vi "DeviceDiscovery.vi"() -> (2 "deviceInfo out":T1, 3 "Ip":string)   [LabVIEW 2019]
uses:
  EmergentCameraC/EmergentCameraC.lvlib
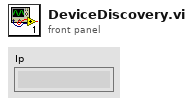
[diagram p1: front panel]
types:
  T1 = cluster{"specVersionMajor":u16, "specVersionMinor":u16, "deviceMode":u32, "macAddress[0]":i8, "macAddress[1]":i8, "macAddress[2]":i8, "macAddress[3]":i8, "macAddress[4]":i8, "macAddress[5]":i8, "macAddress[6]":i8, "macAddress[7]":i8, "macAddress[8]":i8, "macAddress[9]":i8, "macAddress[10]":i8, "macAddress[11]":i8, "macAddress[12]":i8, "macAddress[13]":i8, "macAddress[14]":i8, "macAddress[15]":i8, "macAddress[16]":i8, "macAddress[17]":i8, "@dummy control@":i8, "@dummy control@":i8, "ipConfigOptions":u32, "ipConfigCurrent":u32, "currentIp[0]":i8, "currentIp[1]":i8, "currentIp[2]":i8, "currentIp[3]":i8, "currentIp[4]":i8, "currentIp[5]":i8, "currentIp[6]":i8, "currentIp[7]":i8, "currentIp[8]":i8, "currentIp[9]":i8, "currentIp[10]":i8, "currentIp[11]":i8, "currentIp[12]":i8, "currentIp[13]":i8, "currentIp[14]":i8, "currentIp[15]":i8, "currentSubnetMask[0]":i8, "currentSubnetMask[1]":i8, "currentSubnetMask[2]":i8, "currentSubnetMask[3]":i8, "currentSubnetMask[4]":i8, "currentSubnetMask[5]":i8, "currentSubnetMask[6]":i8, "currentSubnetMask[7]":i8, "currentSubnetMask[8]":i8, "currentSubnetMask[9]":i8, "currentSubnetMask[10]":i8, "currentSubnetMask[11]":i8, "currentSubnetMask[12]":i8, "currentSubnetMask[13]":i8, "currentSubnetMask[14]":i8, "currentSubnetMask[15]":i8, "defaultGateway[0]":i8, "defaultGateway[1]":i8, "defaultGateway[2]":i8, "defaultGateway[3]":i8, "defaultGateway[4]":i8, "defaultGateway[5]":i8, "defaultGateway[6]":i8, "defaultGateway[7]":i8, "defaultGateway[8]":i8, "defaultGateway[9]":i8, "defaultGateway[10]":i8, "defaultGateway[11]":i8, "defaultGateway[12]":i8, "defaultGateway[13]":i8, "defaultGateway[14]":i8, "defaultGateway[15]":i8, "manufacturerName[0]":i8, "manufacturerName[1]":i8, "manufacturerName[2]":i8, "manufacturerName[3]":i8, "manufacturerName[4]":i8, "manufacturerName[5]":i8, "manufacturerName[6]":i8, "manufacturerName[7]":i8, "manufacturerName[8]":i8, "manufacturerName[9]":i8, "manufacturerName[10]":i8, "manufacturerName[11]":i8, "manufacturerName[12]":i8, "manufacturerName[13]":i8, "manufacturerName[14]":i8, "manufacturerName[15]":i8, "manufacturerName[16]":i8, "manufacturerName[17]":i8, "manufacturerName[18]":i8, "manufacturerName[19]":i8, "manufacturerName[20]":i8, "manufacturerName[21]":i8, "manufacturerName[22]":i8, "manufacturerName[23]":i8, "manufacturerName[24]":i8, "manufacturerName[25]":i8, "manufacturerName[26]":i8, "manufacturerName[27]":i8, "manufacturerName[28]":i8, "manufacturerName[29]":i8, "manufacturerName[30]":i8, "manufacturerName[31]":i8, "modelName[0]":i8, "modelName[1]":i8, "modelName[2]":i8, "modelName[3]":i8, "modelName[4]":i8, "modelName[5]":i8, "modelName[6]":i8, "modelName[7]":i8, "modelName[8]":i8, "modelName[9]":i8, "modelName[10]":i8, "modelName[11]":i8, "modelName[12]":i8, "modelName[13]":i8, "modelName[14]":i8, "modelName[15]":i8, "modelName[16]":i8, "modelName[17]":i8, "modelName[18]":i8, "modelName[19]":i8, "modelName[20]":i8, "modelName[21]":i8, "modelName[22]":i8, "modelName[23]":i8, "modelName[24]":i8, "modelName[25]":i8, "modelName[26]":i8, "modelName[27]":i8, "modelName[28]":i8, "modelName[29]":i8, "modelName[30]":i8, "modelName[31]":i8, "deviceVersion[0]":i8, "deviceVersion[1]":i8, "deviceVersion[2]":i8, "deviceVersion[3]":i8, "deviceVersion[4]":i8, "deviceVersion[5]":i8, "deviceVersion[6]":i8, "deviceVersion[7]":i8, "deviceVersion[8]":i8, "deviceVersion[9]":i8, "deviceVersion[10]":i8, "deviceVersion[11]":i8, "deviceVersion[12]":i8, "deviceVersion[13]":i8, "deviceVersion[14]":i8, "deviceVersion[15]":i8, "deviceVersion[16]":i8, "deviceVersion[17]":i8, "deviceVersion[18]":i8, "deviceVersion[19]":i8, "deviceVersion[20]":i8, "deviceVersion[21]":i8, "deviceVersion[22]":i8, "deviceVersion[23]":i8, "deviceVersion[24]":i8, "deviceVersion[25]":i8, "deviceVersion[26]":i8, "deviceVersion[27]":i8, "deviceVersion[28]":i8, "deviceVersion[29]":i8, "deviceVersion[30]":i8, "deviceVersion[31]":i8, "manufacturerSpecifiedInfo[0]":i8, "manufacturerSpecifiedInfo[1]":i8, "manufacturerSpecifiedInfo[2]":i8, "manufacturerSpecifiedInfo[3]":i8, "manufacturerSpecifiedInfo[4]":i8, "manufacturerSpecifiedInfo[5]":i8, "manufacturerSpecifiedInfo[6]":i8, "manufacturerSpecifiedInfo[7]":i8, "manufacturerSpecifiedInfo[8]":i8, "manufacturerSpecifiedInfo[9]":i8, "manufacturerSpecifiedInfo[10]":i8, "manufacturerSpecifiedInfo[11]":i8, "manufacturerSpecifiedInfo[12]":i8, "manufacturerSpecifiedInfo[13]":i8, "manufacturerSpecifiedInfo[14]":i8, "manufacturerSpecifiedInfo[15]":i8, "manufacturerSpecifiedInfo[16]":i8, "manufacturerSpecifiedInfo[17]":i8, "manufacturerSpecifiedInfo[18]":i8, "manufacturerSpecifiedInfo[19]":i8, "manufacturerSpecifiedInfo[20]":i8, "manufacturerSpecifiedInfo[21]":i8, "manufacturerSpecifiedInfo[22]":i8, "manufacturerSpecifiedInfo[23]":i8, "manufacturerSpecifiedInfo[24]":i8, "manufacturerSpecifiedInfo[25]":i8, "manufacturerSpecifiedInfo[26]":i8, "manufacturerSpecifiedInfo[27]":i8, "manufacturerSpecifiedInfo[28]":i8, "manufacturerSpecifiedInfo[29]":i8, "manufacturerSpecifiedInfo[30]":i8, "manufacturerSpecifiedInfo[31]":i8, "manufacturerSpecifiedInfo[32]":i8, "manufacturerSpecifiedInfo[33]":i8, "manufacturerSpecifiedInfo[34]":i8, "manufacturerSpecifiedInfo[35]":i8, "manufacturerSpecifiedInfo[36]":i8, "manufacturerSpecifiedInfo[37]":i8, "manufacturerSpecifiedInfo[38]":i8, "manufacturerSpecifiedInfo[39]":i8, "manufacturerSpecifiedInfo[40]":i8, "manufacturerSpecifiedInfo[41]":i8, "manufacturerSpecifiedInfo[42]":i8, "manufacturerSpecifiedInfo[43]":i8, "manufacturerSpecifiedInfo[44]":i8, "manufacturerSpecifiedInfo[45]":i8, "manufacturerSpecifiedInfo[46]":i8, "manufacturerSpecifiedInfo[47]":i8, "serialNumber[0]":i8, "serialNumber[1]":i8, "serialNumber[2]":i8, "serialNumber[3]":i8, "serialNumber[4]":i8, "serialNumber[5]":i8, "serialNumber[6]":i8, "serialNumber[7]":i8, "serialNumber[8]":i8, "serialNumber[9]":i8, "serialNumber[10]":i8, "serialNumber[11]":i8, "serialNumber[12]":i8, "serialNumber[13]":i8, "serialNumber[14]":i8, "serialNumber[15]":i8, "userDefinedName[0]":i8, "userDefinedName[1]":i8, "userDefinedName[2]":i8, "userDefinedName[3]":i8, "userDefinedName[4]":i8, "userDefinedName[5]":i8, "userDefinedName[6]":i8, "userDefinedName[7]":i8, "userDefinedName[8]":i8, "userDefinedName[9]":i8, "userDefinedName[10]":i8, "userDefinedName[11]":i8, "userDefinedName[12]":i8, "userDefinedName[13]":i8, "userDefinedName[14]":i8, "userDefinedName[15]":i8, "ip4Address[0]":i8, "ip4Address[1]":i8, "ip4Address[2]":i8, "ip4Address[3]":i8, "ip4Address[4]":i8, "ip4Address[5]":i8, "ip4Address[6]":i8, "ip4Address[7]":i8, "ip4Address[8]":i8, "ip4Address[9]":i8, "ip4Address[10]":i8, "ip4Address[11]":i8, "ip4Address[12]":i8, "ip4Address[13]":i8, "ip4Address[14]":i8, "ip4Address[15]":i8, "ip4AddressBroadcast[0]":i8, "ip4AddressBroadcast[1]":i8, "ip4AddressBroadcast[2]":i8, "ip4AddressBroadcast[3]":i8, "ip4AddressBroadcast[4]":i8, "ip4AddressBroadcast[5]":i8, "ip4AddressBroadcast[6]":i8, "ip4AddressBroadcast[7]":i8, "ip4AddressBroadcast[8]":i8, "ip4AddressBroadcast[9]":i8, "ip4AddressBroadcast[10]":i8, "ip4AddressBroadcast[11]":i8, "ip4AddressBroadcast[12]":i8, "ip4AddressBroadcast[13]":i8, "ip4AddressBroadcast[14]":i8, "ip4AddressBroadcast[15]":i8, "friendlyName[0]":i8, "friendlyName[1]":i8, "friendlyName[2]":i8, "friendlyName[3]":i8, "friendlyName[4]":i8, "friendlyName[5]":i8, "friendlyName[6]":i8, "friendlyName[7]":i8, "friendlyName[8]":i8, "friendlyName[9]":i8, "friendlyName[10]":i8, "friendlyName[11]":i8, "friendlyName[12]":i8, "friendlyName[13]":i8, "friendlyName[14]":i8, "friendlyName[15]":i8, "friendlyName[16]":i8, "friendlyName[17]":i8, "friendlyName[18]":i8, "friendlyName[19]":i8, "friendlyName[20]":i8, "friendlyName[21]":i8, "friendlyName[22]":i8, "friendlyName[23]":i8, "friendlyName[24]":i8, "friendlyName[25]":i8, "friendlyName[26]":i8, "friendlyName[27]":i8, "friendlyName[28]":i8, "friendlyName[29]":i8, "friendlyName[30]":i8, "friendlyName[31]":i8, "friendlyName[32]":i8, "friendlyName[33]":i8, "friendlyName[34]":i8, "friendlyName[35]":i8, "friendlyName[36]":i8, "friendlyName[37]":i8, "friendlyName[38]":i8, "friendlyName[39]":i8, "friendlyName[40]":i8, "friendlyName[41]":i8, "friendlyName[42]":i8, "friendlyName[43]":i8, "friendlyName[44]":i8, "friendlyName[45]":i8, "friendlyName[46]":i8, "friendlyName[47]":i8, "friendlyName[48]":i8, "friendlyName[49]":i8, "friendlyName[50]":i8, "friendlyName[51]":i8, "friendlyName[52]":i8, "friendlyName[53]":i8, "friendlyName[54]":i8, "friendlyName[55]":i8, "friendlyName[56]":i8, "friendlyName[57]":i8, "friendlyName[58]":i8, "friendlyName[59]":i8, "friendlyName[60]":i8, "friendlyName[61]":i8, "friendlyName[62]":i8, "friendlyName[63]":i8, "friendlyName[64]":i8, "friendlyName[65]":i8, "friendlyName[66]":i8, "friendlyName[67]":i8, "friendlyName[68]":i8, "friendlyName[69]":i8, "friendlyName[70]":i8, "friendlyName[71]":i8, "friendlyName[72]":i8, "friendlyName[73]":i8, "friendlyName[74]":i8, "friendlyName[75]":i8, "friendlyName[76]":i8, "friendlyName[77]":i8, "friendlyName[78]":i8, "friendlyName[79]":i8, "friendlyName[80]":i8, "friendlyName[81]":i8, "friendlyName[82]":i8, "friendlyName[83]":i8, "friendlyName[84]":i8, "friendlyName[85]":i8, "friendlyName[86]":i8, "friendlyName[87]":i8, "friendlyName[88]":i8, "friendlyName[89]":i8, "friendlyName[90]":i8, "friendlyName[91]":i8, "friendlyName[92]":i8, "friendlyName[93]":i8, "friendlyName[94]":i8, "friendlyName[95]":i8, "friendlyName[96]":i8, "friendlyName[97]":i8, "friendlyName[98]":i8, "friendlyName[99]":i8, "friendlyName[100]":i8, "friendlyName[101]":i8, "friendlyName[102]":i8, "friendlyName[103]":i8, "friendlyName[104]":i8, "friendlyName[105]":i8, "friendlyName[106]":i8, "friendlyName[107]":i8, "friendlyName[108]":i8, "friendlyName[109]":i8, "friendlyName[110]":i8, "friendlyName[111]":i8, "friendlyName[112]":i8, "friendlyName[113]":i8, "friendlyName[114]":i8, "friendlyName[115]":i8, "friendlyName[116]":i8, "friendlyName[117]":i8, "friendlyName[118]":i8, "friendlyName[119]":i8, "friendlyName[120]":i8, "friendlyName[121]":i8, "friendlyName[122]":i8, "friendlyName[123]":i8, "friendlyName[124]":i8, "friendlyName[125]":i8, "friendlyName[126]":i8, "friendlyName[127]":i8, "description[0]":i8, "description[1]":i8, "description[2]":i8, "description[3]":i8, "description[4]":i8, "description[5]":i8, "description[6]":i8, "description[7]":i8, "description[8]":i8, "description[9]":i8, "description[10]":i8, "description[11]":i8, "description[12]":i8, "description[13]":i8, "description[14]":i8, "description[15]":i8, "description[16]":i8, "description[17]":i8, "description[18]":i8, "description[19]":i8, "description[20]":i8, "description[21]":i8, "description[22]":i8, "description[23]":i8, "description[24]":i8, "description[25]":i8, "description[26]":i8, "description[27]":i8, "description[28]":i8, "description[29]":i8, "description[30]":i8, "description[31]":i8, "description[32]":i8, "description[33]":i8, "description[34]":i8, "description[35]":i8, "description[36]":i8, "description[37]":i8, "description[38]":i8, "description[39]":i8, "description[40]":i8, "description[41]":i8, "description[42]":i8, "description[43]":i8, "description[44]":i8, "description[45]":i8, "description[46]":i8, "description[47]":i8, "description[48]":i8, "description[49]":i8, "description[50]":i8, "description[51]":i8, "description[52]":i8, "description[53]":i8, "description[54]":i8, "description[55]":i8, "description[56]":i8, "description[57]":i8, "description[58]":i8, "description[59]":i8, "description[60]":i8, "description[61]":i8, "description[62]":i8, "description[63]":i8, "description[64]":i8, "description[65]":i8, "description[66]":i8, "description[67]":i8, "description[68]":i8, "description[69]":i8, "description[70]":i8, "description[71]":i8, "description[72]":i8, "description[73]":i8, "description[74]":i8, "description[75]":i8, "description[76]":i8, "description[77]":i8, "description[78]":i8, "description[79]":i8, "description[80]":i8, "description[81]":i8, "description[82]":i8, "description[83]":i8, "description[84]":i8, "description[85]":i8, "description[86]":i8, "description[87]":i8, "description[88]":i8, "description[89]":i8, "description[90]":i8, "description[91]":i8, "description[92]":i8, "description[93]":i8, "description[94]":i8, "description[95]":i8, "description[96]":i8, "description[97]":i8, "description[98]":i8, "description[99]":i8, "description[100]":i8, "description[101]":i8, "description[102]":i8, "description[103]":i8, "description[104]":i8, "description[105]":i8, "description[106]":i8, "description[107]":i8, "description[108]":i8, "description[109]":i8, "description[110]":i8, "description[111]":i8, "description[112]":i8, "description[113]":i8, "description[114]":i8, "description[115]":i8, "description[116]":i8, "description[117]":i8, "description[118]":i8, "description[119]":i8, "description[120]":i8, "description[121]":i8, "description[122]":i8, "description[123]":i8, "description[124]":i8, "description[125]":i8, "description[126]":i8, "description[127]":i8, "adapterName[0]":i8, "adapterName[1]":i8, "adapterName[2]":i8, "adapterName[3]":i8, "adapterName[4]":i8, "adapterName[5]":i8, "adapterName[6]":i8, "adapterName[7]":i8, "adapterName[8]":i8, "adapterName[9]":i8, "adapterName[10]":i8, "adapterName[11]":i8, "adapterName[12]":i8, "adapterName[13]":i8, "adapterName[14]":i8, "adapterName[15]":i8, "adapterName[16]":i8, "adapterName[17]":i8, "adapterName[18]":i8, "adapterName[19]":i8, "adapterName[20]":i8, "adapterName[21]":i8, "adapterName[22]":i8, "adapterName[23]":i8, "adapterName[24]":i8, "adapterName[25]":i8, "adapterName[26]":i8, "adapterName[27]":i8, "adapterName[28]":i8, "adapterName[29]":i8, "adapterName[30]":i8, "adapterName[31]":i8, "adapterName[32]":i8, "adapterName[33]":i8, "adapterName[34]":i8, "adapterName[35]":i8, "adapterName[36]":i8, "adapterName[37]":i8, "adapterName[38]":i8, "adapterName[39]":i8, "adapterName[40]":i8, "adapterName[41]":i8, "adapterName[42]":i8, "adapterName[43]":i8, "adapterName[44]":i8, "adapterName[45]":i8, "adapterName[46]":i8, "adapterName[47]":i8, "adapterName[48]":i8, "adapterName[49]":i8, "adapterName[50]":i8, "adapterName[51]":i8, "adapterName[52]":i8, "adapterName[53]":i8, "adapterName[54]":i8, "adapterName[55]":i8, "adapterName[56]":i8, "adapterName[57]":i8, "adapterName[58]":i8, "adapterName[59]":i8, "adapterName[60]":i8, "adapterName[61]":i8, "adapterName[62]":i8, "adapterName[63]":i8, "adapterName[64]":i8, "adapterName[65]":i8, "adapterName[66]":i8, "adapterName[67]":i8, "adapterName[68]":i8, "adapterName[69]":i8, "adapterName[70]":i8, "adapterName[71]":i8, "adapterName[72]":i8, "adapterName[73]":i8, "adapterName[74]":i8, "adapterName[75]":i8, "adapterName[76]":i8, "adapterName[77]":i8, "adapterName[78]":i8, "adapterName[79]":i8, "adapterName[80]":i8, "adapterName[81]":i8, "adapterName[82]":i8, "adapterName[83]":i8, "adapterName[84]":i8, "adapterName[85]":i8, "adapterName[86]":i8, "adapterName[87]":i8, "adapterName[88]":i8, "adapterName[89]":i8, "adapterName[90]":i8, "adapterName[91]":i8, "adapterName[92]":i8, "adapterName[93]":i8, "adapterName[94]":i8, "adapterName[95]":i8, "adapterName[96]":i8, "adapterName[97]":i8, "adapterName[98]":i8, "adapterName[99]":i8, "adapterName[100]":i8, "adapterName[101]":i8, "adapterName[102]":i8, "adapterName[103]":i8, "adapterName[104]":i8, "adapterName[105]":i8, "adapterName[106]":i8, "adapterName[107]":i8, "adapterName[108]":i8, "adapterName[109]":i8, "adapterName[110]":i8, "adapterName[111]":i8, "adapterName[112]":i8, "adapterName[113]":i8, "adapterName[114]":i8, "adapterName[115]":i8, "adapterName[116]":i8, "adapterName[117]":i8, "adapterName[118]":i8, "adapterName[119]":i8, "adapterName[120]":i8, "adapterName[121]":i8, "adapterName[122]":i8, "adapterName[123]":i8, "adapterName[124]":i8, "adapterName[125]":i8, "adapterName[126]":i8, "adapterName[127]":i8, "vendorID":u32, "@dummy control@":i8, "@dummy control@":i8, "@dummy control@":i8, "@dummy control@":i8, "@dummy control@":i8, "@dummy control@":i8, "@dummy control@":i8, "@dummy control@":i8, "name":u64, "fullName":u64, "mtu":u32}
  T2 = cluster{"currentIp[0]":i8, "currentIp[1]":i8, "currentIp[2]":i8, "currentIp[3]":i8, "currentIp[4]":i8, "currentIp[5]":i8, "currentIp[6]":i8, "currentIp[7]":i8, "currentIp[8]":i8, "currentIp[9]":i8, "currentIp[10]":i8, "currentIp[11]":i8, "currentIp[12]":i8, "currentIp[13]":i8, "currentIp[14]":i8, "currentIp[15]":i8}
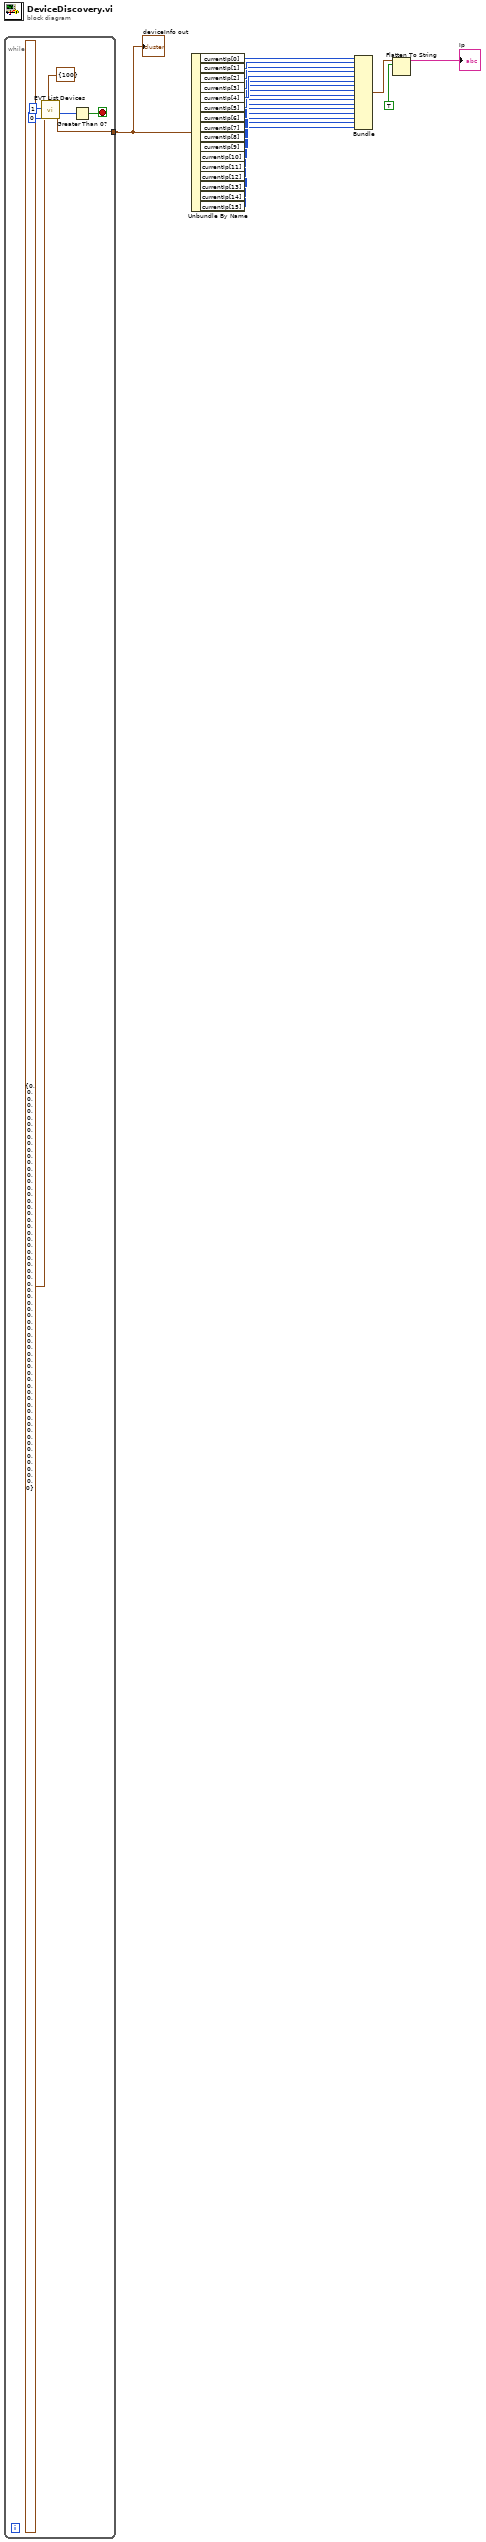
[diagram p0: block diagram]
diagram:
  n1 = while {
    tunnel: [w24] -> w2
    stop <- w23 stop-if-true
    n2 = call "EVT List Devices.vi"("settings"=cluster{"timeout":i32} {"timeout"=100}, "actualNum"=u32 0, "bufSize"=u32 1, "deviceInfo"=T1 {"specVersionMajor"=0, "specVersionMinor"=0, "deviceMode"=0, "macAddress[0]"=0, "macAddress[1]"=0, "macAddress[2]"=0, "macAddress[3]"=0, "macAddress[4]"=0, "macAddress[5]"=0, "macAddress[6]"=0, "macAddress[7]"=0, "macAddress[8]"=0, "macAddress[9]"=0, "macAddress[10]"=0, "macAddress[11]"=0, "macAddress[12]"=0, "macAddress[13]"=0, "macAddress[14]"=0, "macAddress[15]"=0, "macAddress[16]"=0, "macAddress[17]"=0, "@dummy control@"=0, "@dummy control@"=0, "ipConfigOptions"=0, "ipConfigCurrent"=0, "currentIp[0]"=0, "currentIp[1]"=0, "currentIp[2]"=0, "currentIp[3]"=0, "currentIp[4]"=0, "currentIp[5]"=0, "currentIp[6]"=0, "currentIp[7]"=0, "currentIp[8]"=0, "currentIp[9]"=0, "currentIp[10]"=0, "currentIp[11]"=0, "currentIp[12]"=0, "currentIp[13]"=0, "currentIp[14]"=0, "currentIp[15]"=0, "currentSubnetMask[0]"=0, "currentSubnetMask[1]"=0, "currentSubnetMask[2]"=0, "currentSubnetMask[3]"=0, "currentSubnetMask[4]"=0, "currentSubnetMask[5]"=0, "currentSubnetMask[6]"=0, "currentSubnetMask[7]"=0, "currentSubnetMask[8]"=0, "currentSubnetMask[9]"=0, "currentSubnetMask[10]"=0, "currentSubnetMask[11]"=0, "currentSubnetMask[12]"=0, "currentSubnetMask[13]"=0, "currentSubnetMask[14]"=0, "currentSubnetMask[15]"=0, "defaultGateway[0]"=0, "defaultGateway[1]"=0, "defaultGateway[2]"=0, "defaultGateway[3]"=0, "defaultGateway[4]"=0, "defaultGateway[5]"=0, "defaultGateway[6]"=0, "defaultGateway[7]"=0, "defaultGateway[8]"=0, "defaultGateway[9]"=0, "defaultGateway[10]"=0, "defaultGateway[11]"=0, "defaultGateway[12]"=0, "defaultGateway[13]"=0, "defaultGateway[14]"=0, "defaultGateway[15]"=0, "manufacturerName[0]"=0, "manufacturerName[1]"=0, "manufacturerName[2]"=0, "manufacturerName[3]"=0, "manufacturerName[4]"=0, "manufacturerName[5]"=0, "manufacturerName[6]"=0, "manufacturerName[7]"=0, "manufacturerName[8]"=0, "manufacturerName[9]"=0, "manufacturerName[10]"=0, "manufacturerName[11]"=0, "manufacturerName[12]"=0, "manufacturerName[13]"=0, "manufacturerName[14]"=0, "manufacturerName[15]"=0, "manufacturerName[16]"=0, "manufacturerName[17]"=0, "manufacturerName[18]"=0, "manufacturerName[19]"=0, "manufacturerName[20]"=0, "manufacturerName[21]"=0, "manufacturerName[22]"=0, "manufacturerName[23]"=0, "manufacturerName[24]"=0, "manufacturerName[25]"=0, "manufacturerName[26]"=0, "manufacturerName[27]"=0, "manufacturerName[28]"=0, "manufacturerName[29]"=0, "manufacturerName[30]"=0, "manufacturerName[31]"=0, "modelName[0]"=0, "modelName[1]"=0, "modelName[2]"=0, "modelName[3]"=0, "modelName[4]"=0, "modelName[5]"=0, "modelName[6]"=0, "modelName[7]"=0, "modelName[8]"=0, "modelName[9]"=0, "modelName[10]"=0, "modelName[11]"=0, "modelName[12]"=0, "modelName[13]"=0, "modelName[14]"=0, "modelName[15]"=0, "modelName[16]"=0, "modelName[17]"=0, "modelName[18]"=0, "modelName[19]"=0, "modelName[20]"=0, "modelName[21]"=0, "modelName[22]"=0, "modelName[23]"=0, "modelName[24]"=0, "modelName[25]"=0, "modelName[26]"=0, "modelName[27]"=0, "modelName[28]"=0, "modelName[29]"=0, "modelName[30]"=0, "modelName[31]"=0, "deviceVersion[0]"=0, "deviceVersion[1]"=0, "deviceVersion[2]"=0, "deviceVersion[3]"=0, "deviceVersion[4]"=0, "deviceVersion[5]"=0, "deviceVersion[6]"=0, "deviceVersion[7]"=0, "deviceVersion[8]"=0, "deviceVersion[9]"=0, "deviceVersion[10]"=0, "deviceVersion[11]"=0, "deviceVersion[12]"=0, "deviceVersion[13]"=0, "deviceVersion[14]"=0, "deviceVersion[15]"=0, "deviceVersion[16]"=0, "deviceVersion[17]"=0, "deviceVersion[18]"=0, "deviceVersion[19]"=0, "deviceVersion[20]"=0, "deviceVersion[21]"=0, "deviceVersion[22]"=0, "deviceVersion[23]"=0, "deviceVersion[24]"=0, "deviceVersion[25]"=0, "deviceVersion[26]"=0, "deviceVersion[27]"=0, "deviceVersion[28]"=0, "deviceVersion[29]"=0, "deviceVersion[30]"=0, "deviceVersion[31]"=0, "manufacturerSpecifiedInfo[0]"=0, "manufacturerSpecifiedInfo[1]"=0, "manufacturerSpecifiedInfo[2]"=0, "manufacturerSpecifiedInfo[3]"=0, "manufacturerSpecifiedInfo[4]"=0, "manufacturerSpecifiedInfo[5]"=0, "manufacturerSpecifiedInfo[6]"=0, "manufacturerSpecifiedInfo[7]"=0, "manufacturerSpecifiedInfo[8]"=0, "manufacturerSpecifiedInfo[9]"=0, "manufacturerSpecifiedInfo[10]"=0, "manufacturerSpecifiedInfo[11]"=0, "manufacturerSpecifiedInfo[12]"=0, "manufacturerSpecifiedInfo[13]"=0, "manufacturerSpecifiedInfo[14]"=0, "manufacturerSpecifiedInfo[15]"=0, "manufacturerSpecifiedInfo[16]"=0, "manufacturerSpecifiedInfo[17]"=0, "manufacturerSpecifiedInfo[18]"=0, "manufacturerSpecifiedInfo[19]"=0, "manufacturerSpecifiedInfo[20]"=0, "manufacturerSpecifiedInfo[21]"=0, "manufacturerSpecifiedInfo[22]"=0, "manufacturerSpecifiedInfo[23]"=0, "manufacturerSpecifiedInfo[24]"=0, "manufacturerSpecifiedInfo[25]"=0, "manufacturerSpecifiedInfo[26]"=0, "manufacturerSpecifiedInfo[27]"=0, "manufacturerSpecifiedInfo[28]"=0, "manufacturerSpecifiedInfo[29]"=0, "manufacturerSpecifiedInfo[30]"=0, "manufacturerSpecifiedInfo[31]"=0, "manufacturerSpecifiedInfo[32]"=0, "manufacturerSpecifiedInfo[33]"=0, "manufacturerSpecifiedInfo[34]"=0, "manufacturerSpecifiedInfo[35]"=0, "manufacturerSpecifiedInfo[36]"=0, "manufacturerSpecifiedInfo[37]"=0, "manufacturerSpecifiedInfo[38]"=0, "manufacturerSpecifiedInfo[39]"=0, "manufacturerSpecifiedInfo[40]"=0, "manufacturerSpecifiedInfo[41]"=0, "manufacturerSpecifiedInfo[42]"=0, "manufacturerSpecifiedInfo[43]"=0, "manufacturerSpecifiedInfo[44]"=0, "manufacturerSpecifiedInfo[45]"=0, "manufacturerSpecifiedInfo[46]"=0, "manufacturerSpecifiedInfo[47]"=0, "serialNumber[0]"=0, "serialNumber[1]"=0, "serialNumber[2]"=0, "serialNumber[3]"=0, "serialNumber[4]"=0, "serialNumber[5]"=0, "serialNumber[6]"=0, "serialNumber[7]"=0, "serialNumber[8]"=0, "serialNumber[9]"=0, "serialNumber[10]"=0, "serialNumber[11]"=0, "serialNumber[12]"=0, "serialNumber[13]"=0, "serialNumber[14]"=0, "serialNumber[15]"=0, "userDefinedName[0]"=0, "userDefinedName[1]"=0, "userDefinedName[2]"=0, "userDefinedName[3]"=0, "userDefinedName[4]"=0, "userDefinedName[5]"=0, "userDefinedName[6]"=0, "userDefinedName[7]"=0, "userDefinedName[8]"=0, "userDefinedName[9]"=0, "userDefinedName[10]"=0, "userDefinedName[11]"=0, "userDefinedName[12]"=0, "userDefinedName[13]"=0, "userDefinedName[14]"=0, "userDefinedName[15]"=0, "ip4Address[0]"=0, "ip4Address[1]"=0, "ip4Address[2]"=0, "ip4Address[3]"=0, "ip4Address[4]"=0, "ip4Address[5]"=0, "ip4Address[6]"=0, "ip4Address[7]"=0, "ip4Address[8]"=0, "ip4Address[9]"=0, "ip4Address[10]"=0, "ip4Address[11]"=0, "ip4Address[12]"=0, "ip4Address[13]"=0, "ip4Address[14]"=0, "ip4Address[15]"=0, "ip4AddressBroadcast[0]"=0, "ip4AddressBroadcast[1]"=0, "ip4AddressBroadcast[2]"=0, "ip4AddressBroadcast[3]"=0, "ip4AddressBroadcast[4]"=0, "ip4AddressBroadcast[5]"=0, "ip4AddressBroadcast[6]"=0, "ip4AddressBroadcast[7]"=0, "ip4AddressBroadcast[8]"=0, "ip4AddressBroadcast[9]"=0, "ip4AddressBroadcast[10]"=0, "ip4AddressBroadcast[11]"=0, "ip4AddressBroadcast[12]"=0, "ip4AddressBroadcast[13]"=0, "ip4AddressBroadcast[14]"=0, "ip4AddressBroadcast[15]"=0, "friendlyName[0]"=0, "friendlyName[1]"=0, "friendlyName[2]"=0, "friendlyName[3]"=0, "friendlyName[4]"=0, "friendlyName[5]"=0, "friendlyName[6]"=0, "friendlyName[7]"=0, "friendlyName[8]"=0, "friendlyName[9]"=0, "friendlyName[10]"=0, "friendlyName[11]"=0, "friendlyName[12]"=0, "friendlyName[13]"=0, "friendlyName[14]"=0, "friendlyName[15]"=0, "friendlyName[16]"=0, "friendlyName[17]"=0, "friendlyName[18]"=0, "friendlyName[19]"=0, "friendlyName[20]"=0, "friendlyName[21]"=0, "friendlyName[22]"=0, "friendlyName[23]"=0, "friendlyName[24]"=0, "friendlyName[25]"=0, "friendlyName[26]"=0, "friendlyName[27]"=0, "friendlyName[28]"=0, "friendlyName[29]"=0, "friendlyName[30]"=0, "friendlyName[31]"=0, "friendlyName[32]"=0, "friendlyName[33]"=0, "friendlyName[34]"=0, "friendlyName[35]"=0, "friendlyName[36]"=0, "friendlyName[37]"=0, "friendlyName[38]"=0, "friendlyName[39]"=0, "friendlyName[40]"=0, "friendlyName[41]"=0, "friendlyName[42]"=0, "friendlyName[43]"=0, "friendlyName[44]"=0, "friendlyName[45]"=0, "friendlyName[46]"=0, "friendlyName[47]"=0, "friendlyName[48]"=0, "friendlyName[49]"=0, "friendlyName[50]"=0, "friendlyName[51]"=0, "friendlyName[52]"=0, "friendlyName[53]"=0, "friendlyName[54]"=0, "friendlyName[55]"=0, "friendlyName[56]"=0, "friendlyName[57]"=0, "friendlyName[58]"=0, "friendlyName[59]"=0, "friendlyName[60]"=0, "friendlyName[61]"=0, "friendlyName[62]"=0, "friendlyName[63]"=0, "friendlyName[64]"=0, "friendlyName[65]"=0, "friendlyName[66]"=0, "friendlyName[67]"=0, "friendlyName[68]"=0, "friendlyName[69]"=0, "friendlyName[70]"=0, "friendlyName[71]"=0, "friendlyName[72]"=0, "friendlyName[73]"=0, "friendlyName[74]"=0, "friendlyName[75]"=0, "friendlyName[76]"=0, "friendlyName[77]"=0, "friendlyName[78]"=0, "friendlyName[79]"=0, "friendlyName[80]"=0, "friendlyName[81]"=0, "friendlyName[82]"=0, "friendlyName[83]"=0, "friendlyName[84]"=0, "friendlyName[85]"=0, "friendlyName[86]"=0, "friendlyName[87]"=0, "friendlyName[88]"=0, "friendlyName[89]"=0, "friendlyName[90]"=0, "friendlyName[91]"=0, "friendlyName[92]"=0, "friendlyName[93]"=0, "friendlyName[94]"=0, "friendlyName[95]"=0, "friendlyName[96]"=0, "friendlyName[97]"=0, "friendlyName[98]"=0, "friendlyName[99]"=0, "friendlyName[100]"=0, "friendlyName[101]"=0, "friendlyName[102]"=0, "friendlyName[103]"=0, "friendlyName[104]"=0, "friendlyName[105]"=0, "friendlyName[106]"=0, "friendlyName[107]"=0, "friendlyName[108]"=0, "friendlyName[109]"=0, "friendlyName[110]"=0, "friendlyName[111]"=0, "friendlyName[112]"=0, "friendlyName[113]"=0, "friendlyName[114]"=0, "friendlyName[115]"=0, "friendlyName[116]"=0, "friendlyName[117]"=0, "friendlyName[118]"=0, "friendlyName[119]"=0, "friendlyName[120]"=0, "friendlyName[121]"=0, "friendlyName[122]"=0, "friendlyName[123]"=0, "friendlyName[124]"=0, "friendlyName[125]"=0, "friendlyName[126]"=0, "friendlyName[127]"=0, "description[0]"=0, "description[1]"=0, "description[2]"=0, "description[3]"=0, "description[4]"=0, "description[5]"=0, "description[6]"=0, "description[7]"=0, "description[8]"=0, "description[9]"=0, "description[10]"=0, "description[11]"=0, "description[12]"=0, "description[13]"=0, "description[14]"=0, "description[15]"=0, "description[16]"=0, "description[17]"=0, "description[18]"=0, "description[19]"=0, "description[20]"=0, "description[21]"=0, "description[22]"=0, "description[23]"=0, "description[24]"=0, "description[25]"=0, "description[26]"=0, "description[27]"=0, "description[28]"=0, "description[29]"=0, "description[30]"=0, "description[31]"=0, "description[32]"=0, "description[33]"=0, "description[34]"=0, "description[35]"=0, "description[36]"=0, "description[37]"=0, "description[38]"=0, "description[39]"=0, "description[40]"=0, "description[41]"=0, "description[42]"=0, "description[43]"=0, "description[44]"=0, "description[45]"=0, "description[46]"=0, "description[47]"=0, "description[48]"=0, "description[49]"=0, "description[50]"=0, "description[51]"=0, "description[52]"=0, "description[53]"=0, "description[54]"=0, "description[55]"=0, "description[56]"=0, "description[57]"=0, "description[58]"=0, "description[59]"=0, "description[60]"=0, "description[61]"=0, "description[62]"=0, "description[63]"=0, "description[64]"=0, "description[65]"=0, "description[66]"=0, "description[67]"=0, "description[68]"=0, "description[69]"=0, "description[70]"=0, "description[71]"=0, "description[72]"=0, "description[73]"=0, "description[74]"=0, "description[75]"=0, "description[76]"=0, "description[77]"=0, "description[78]"=0, "description[79]"=0, "description[80]"=0, "description[81]"=0, "description[82]"=0, "description[83]"=0, "description[84]"=0, "description[85]"=0, "description[86]"=0, "description[87]"=0, "description[88]"=0, "description[89]"=0, "description[90]"=0, "description[91]"=0, "description[92]"=0, "description[93]"=0, "description[94]"=0, "description[95]"=0, "description[96]"=0, "description[97]"=0, "description[98]"=0, "description[99]"=0, "description[100]"=0, "description[101]"=0, "description[102]"=0, "description[103]"=0, "description[104]"=0, "description[105]"=0, "description[106]"=0, "description[107]"=0, "description[108]"=0, "description[109]"=0, "description[110]"=0, "description[111]"=0, "description[112]"=0, "description[113]"=0, "description[114]"=0, "description[115]"=0, "description[116]"=0, "description[117]"=0, "description[118]"=0, "description[119]"=0, "description[120]"=0, "description[121]"=0, "description[122]"=0, "description[123]"=0, "description[124]"=0, "description[125]"=0, "description[126]"=0, "description[127]"=0, "adapterName[0]"=0, "adapterName[1]"=0, "adapterName[2]"=0, "adapterName[3]"=0, "adapterName[4]"=0, "adapterName[5]"=0, "adapterName[6]"=0, "adapterName[7]"=0, "adapterName[8]"=0, "adapterName[9]"=0, "adapterName[10]"=0, "adapterName[11]"=0, "adapterName[12]"=0, "adapterName[13]"=0, "adapterName[14]"=0, "adapterName[15]"=0, "adapterName[16]"=0, "adapterName[17]"=0, "adapterName[18]"=0, "adapterName[19]"=0, "adapterName[20]"=0, "adapterName[21]"=0, "adapterName[22]"=0, "adapterName[23]"=0, "adapterName[24]"=0, "adapterName[25]"=0, "adapterName[26]"=0, "adapterName[27]"=0, "adapterName[28]"=0, "adapterName[29]"=0, "adapterName[30]"=0, "adapterName[31]"=0, "adapterName[32]"=0, "adapterName[33]"=0, "adapterName[34]"=0, "adapterName[35]"=0, "adapterName[36]"=0, "adapterName[37]"=0, "adapterName[38]"=0, "adapterName[39]"=0, "adapterName[40]"=0, "adapterName[41]"=0, "adapterName[42]"=0, "adapterName[43]"=0, "adapterName[44]"=0, "adapterName[45]"=0, "adapterName[46]"=0, "adapterName[47]"=0, "adapterName[48]"=0, "adapterName[49]"=0, "adapterName[50]"=0, "adapterName[51]"=0, "adapterName[52]"=0, "adapterName[53]"=0, "adapterName[54]"=0, "adapterName[55]"=0, "adapterName[56]"=0, "adapterName[57]"=0, "adapterName[58]"=0, "adapterName[59]"=0, "adapterName[60]"=0, "adapterName[61]"=0, "adapterName[62]"=0, "adapterName[63]"=0, "adapterName[64]"=0, "adapterName[65]"=0, "adapterName[66]"=0, "adapterName[67]"=0, "adapterName[68]"=0, "adapterName[69]"=0, "adapterName[70]"=0, "adapterName[71]"=0, "adapterName[72]"=0, "adapterName[73]"=0, "adapterName[74]"=0, "adapterName[75]"=0, "adapterName[76]"=0, "adapterName[77]"=0, "adapterName[78]"=0, "adapterName[79]"=0, "adapterName[80]"=0, "adapterName[81]"=0, "adapterName[82]"=0, "adapterName[83]"=0, "adapterName[84]"=0, "adapterName[85]"=0, "adapterName[86]"=0, "adapterName[87]"=0, "adapterName[88]"=0, "adapterName[89]"=0, "adapterName[90]"=0, "adapterName[91]"=0, "adapterName[92]"=0, "adapterName[93]"=0, "adapterName[94]"=0, "adapterName[95]"=0, "adapterName[96]"=0, "adapterName[97]"=0, "adapterName[98]"=0, "adapterName[99]"=0, "adapterName[100]"=0, "adapterName[101]"=0, "adapterName[102]"=0, "adapterName[103]"=0, "adapterName[104]"=0, "adapterName[105]"=0, "adapterName[106]"=0, "adapterName[107]"=0, "adapterName[108]"=0, "adapterName[109]"=0, "adapterName[110]"=0, "adapterName[111]"=0, "adapterName[112]"=0, "adapterName[113]"=0, "adapterName[114]"=0, "adapterName[115]"=0, "adapterName[116]"=0, "adapterName[117]"=0, "adapterName[118]"=0, "adapterName[119]"=0, "adapterName[120]"=0, "adapterName[121]"=0, "adapterName[122]"=0, "adapterName[123]"=0, "adapterName[124]"=0, "adapterName[125]"=0, "adapterName[126]"=0, "adapterName[127]"=0, "vendorID"=0, "@dummy control@"=0, "@dummy control@"=0, "@dummy control@"=0, "@dummy control@"=0, "@dummy control@"=0, "@dummy control@"=0, "@dummy control@"=0, "@dummy control@"=0, "name"=0, "fullName"=0, "mtu"=0}) -> ("actualNum out"=w25:u32, "deviceInfo out"=w24:T1)  [unwired: 2 in, 4 out]
    n3 = Greater Than 0?(x=w25) -> (x > 0?=w23:bool)
  }
  "deviceInfo out" <- w2
  n4 = Unbundle By Name(w2) -> ("currentIp[0]"=w18:i8, "currentIp[1]"=w17:i8, "currentIp[2]"=w16:i8, "currentIp[3]"=w15:i8, "currentIp[4]"=w14:i8, "currentIp[5]"=w13:i8, "currentIp[6]"=w12:i8, "currentIp[7]"=w11:i8, "currentIp[8]"=w10:i8, "currentIp[9]"=w9:i8, "currentIp[10]"=w8:i8, "currentIp[11]"=w7:i8, "currentIp[12]"=w6:i8, "currentIp[13]"=w5:i8, "currentIp[14]"=w4:i8, "currentIp[15]"=w3:i8)
  n5 = Bundle "Bundle"("currentIp[0]"=w18, "currentIp[1]"=w17, "currentIp[2]"=w16, "currentIp[3]"=w15, "currentIp[4]"=w14, "currentIp[5]"=w13, "currentIp[6]"=w12, "currentIp[7]"=w11, "currentIp[8]"=w10, "currentIp[9]"=w9, "currentIp[10]"=w8, "currentIp[11]"=w7, "currentIp[12]"=w6, "currentIp[13]"=w5, "currentIp[14]"=w4, "currentIp[15]"=w3) -> (w20:T2)  [unwired: 1 in]
  n6 = Flatten To String(anything=w20, prepend array or string size? (T)=TRUE) -> (data string=→"Ip":string)  [unwired: 2 in, 2 out]
